vi "MongoDB.Database.AddUser.vi"(8 "error in (no error)":errorcluster, 11 "MongoDB.Database in":refnum<class "MongoDB.Database.lvclass">) -> (0 "error out":errorcluster, 3 "MongoDB.Database out":refnum<class "MongoDB.Database.lvclass">)   [LabVIEW 2014, in "MongoDB.Database.lvclass"]
uses:
  MongoDB.Database.lvclass
  C:/MongoData/Drivers/mongo-csharp-driver-2.0.0-beta4/mongo-csharp-driver-2.0.0-beta4/src/MongoDB.Driver.Legacy/bin/Release/MongoDB.Driver.Legacy.dll
  src/MongoDB.Driver.Legacy/bin/Release/MongoDB.Driver.Legacy.dll
  MongoDB.Database.lvclass/MongoDB.Database.ctl
panel:
  in  "user":refnum<k24>
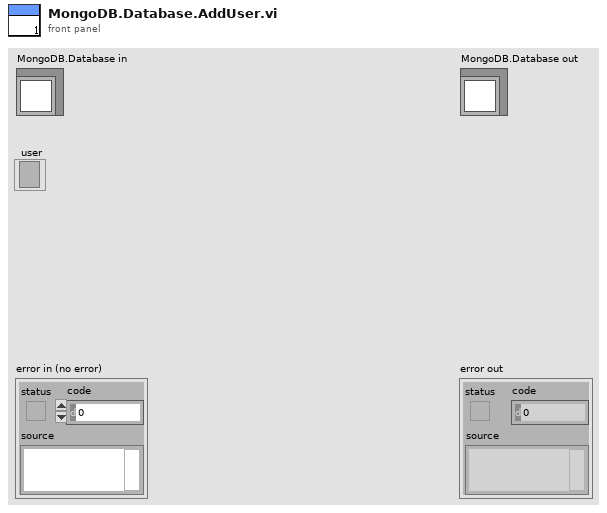
[diagram p1: front panel]
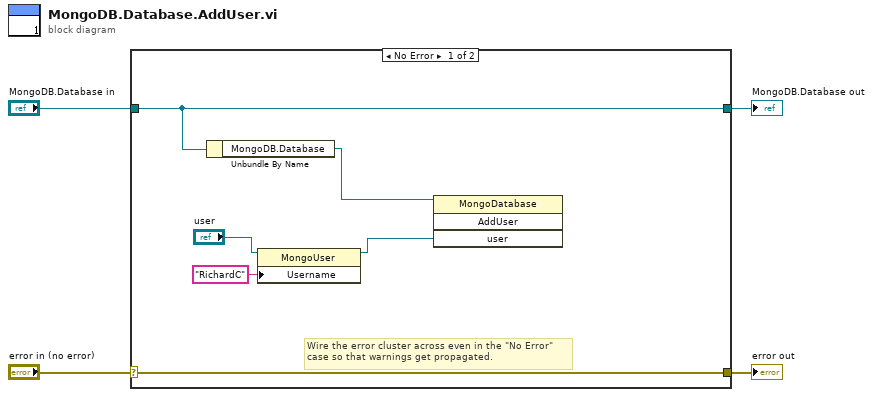
[diagram p0: block diagram]
diagram:
  n1 = case shown="No Error" "error in (no error)" {
    selector: "error in (no error)" -> [w10 w12]
    tunnel: [w10 w12] -> w3
    tunnel: [w9 w11] -> w1
    tunnel: "MongoDB.Database in" -> [w9 w11]
    frame No Error {
      # "Wire the error cluster across even in the \"No Error\"\ncase so that warnings get propagated."
      n2 = Unbundle By Name(w9) -> ("MongoDB.Database"=w8:refnum<k24>)
      n3 = property class="MongoUser"(reference="user", "Username"="RichardC") -> (reference out=w5:refnum<k24>)  [unwired: 1 in, 1 out]
      n4 = invoke class="MongoDatabase" method="AddUser"(reference=w8, "user"=w5) -> ()  [unwired: 2 in, 4 out]
    }
    frame Error {
    }
  }
  "error out" <- w3
  "MongoDB.Database out" <- w1
